vi "Stop.vi"(8 "error in (no error)":errorcluster, 10 "Message in":refnum<class "StopMessage.lvclass">, 11 "Cascade in":refnum<class "Cascade.lvclass">) -> (0 "error out":errorcluster, 3 "Cascade out":refnum<class "Cascade.lvclass">)   [LabVIEW 2012, in "Cascade.lvclass"]
doc: "This member function is called when the statemachine in the run.vi receives an 'stop' command. It relays the message to all observers of the component.\n\nOverride this member function in your derived class if you need additional stop functionality (but don't forget to call the parent method)."
uses:
  Cascade.lvclass
  <vilib>/Distrio/Murmex/Murmex/Murmex.lvclass
  <vilib>/Distrio/Murmex/StopMessage/StopMessage.lvclass
panel:
  # "This method is called when the STOP\ntrigger is sent. \n\nOverride this method when your component needs to\nrespond to this trigger. \n\nCall parent for proper implementation"
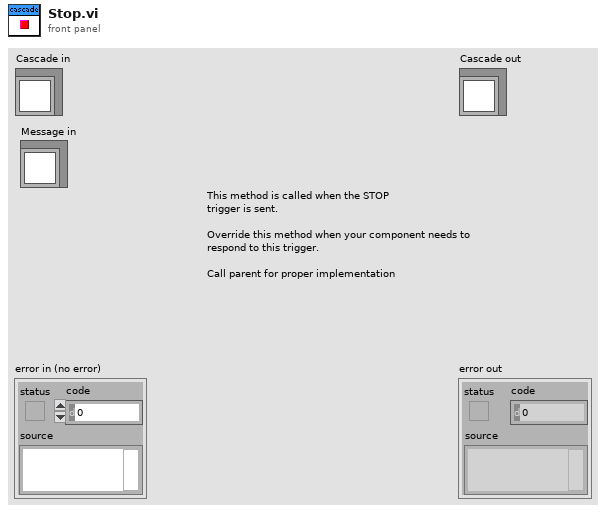
[diagram p1: front panel]
types:
  T1 = enum8{"Enabled", "Disabled", "Disabled and Grayed Out"}
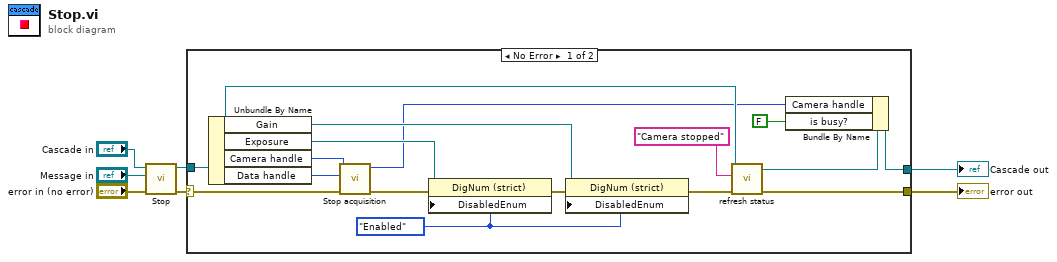
[diagram p0: block diagram]
diagram:
  n1 = call-parent "Stop.vi"("error in (no error)"="error in (no error)", "Message in"="Message in", "Murmex in"="Cascade in") -> ("error out"=w1:errorcluster, "Murmex out"=w2:refnum<class "Cascade.lvclass">)  [unwired: 7 in]
  n2 = case shown="No Error" w1 {
    selector: w1 -> [w12 w24]
    tunnel: w2 -> [w20 w25]
    tunnel: [w21 w24] -> w4
    tunnel: [w23 w25] -> w3
    frame No Error {
      w13 = T1."Enabled" ("Disabled")
      n3 = Unbundle By Name(w20) -> ("Gain"=w14:refnum<vi>, "Exposure"=w15:refnum<vi>, "Camera handle"=w9:i16, "Data handle"=w10:i32)
      n4 = call "Stop acquisition.vi"("error in (no error)"=w12, "buffer ref"=w10, "camera handle in"=w9) -> ("error out"=w11:errorcluster, "camera handle out"=w8:i16)  [unwired: 7 in]
      n5 = property class="DigNum (strict)"(reference=w15, error in=w11, "DisabledEnum"=w13) -> (error out=w17:errorcluster)  [unwired: 1 out]
      n6 = property class="DigNum (strict)"(reference=w14, error in=w17, "DisabledEnum"=w13) -> (error out=w16:errorcluster)  [unwired: 1 out]
      n7 = call-dynamic "refresh status.vi"("error in (no error)"=w16, "String In"="Camera stopped", "Cascade in"=w20) -> ("error out"=w21:errorcluster, "Cascade out"=w19:refnum<class "Cascade.lvclass">)  [unwired: 7 in]
      n8 = Bundle By Name(cluster=w19, "Camera handle"=w8, "is busy?"=FALSE ("runtime.is busy?")) -> (w23:refnum<class "Cascade.lvclass">)
    }
    frame Error {
    }
  }
  "error out" <- w4
  "Cascade out" <- w3
